vi "SMU Switch Handshaking - Advanced - DMM- RT.vi"(8 "error in":errorcluster, 11 "file path (use dialog)":path=path "C:/jsontestfile.json") -> (0 "error out":errorcluster, 2 "Results":T1)   [LabVIEW 2019]
uses:
  <instrlib>/niSwitch/niSwitch.llb/niSwitch Topologies.ctl
  <instrlib>/niSwitch/niSwitch.llb/niSwitch Trigger Input.ctl
  <instrlib>/niSwitch/niSwitch.llb/niSwitch Scan Advanced Output.ctl
  <instrlib>/niDMM/nidmm.llb/niDMM Function.ctl
  <instrlib>/niDMM/nidmm.llb/niDMM Trigger.ctl
  <instrlib>/niDMM/nidmm.llb/niDMM Slope.ctl
  Results.ctl
  <instrlib>/niDCPower/nidcpower.llb/niDCPower Export Signal - Signal.ctl
  <instrlib>/niDMM/nidmm.llb/niDMM Sample Trigger.ctl
  <instrlib>/niDMM/nidmm.llb/niDMM Control Actions.ctl
  <instrlib>/niDCPower/nidcpower.llb/niDCPower Wait For Event - Event.ctl
  <instrlib>/niDMM/nidmm.llb/niDMM Configure Measurement Absolute.vi
  <instrlib>/niDCPower/nidcpower.llb/niDCPower Configure Digital Edge Start Trigger.vi
  <instrlib>/niDCPower/nidcpower.llb/niDCPower Configure Digital Edge Sequence Advance Trigger.vi
  <vilib>/ptbypt/NI_PtbyPt.lvlib
panel:
  out "Results":dbl[][](array[numeric])
  out "R ch5 Array":dbl[](array[numeric])
  out "R ch4 Array":dbl[](array[numeric])
  out "R ch3 Array":dbl[](array[numeric])
  out "R ch2 Array":dbl[](array[numeric])
  out "R ch1 Array":dbl[](array[numeric])
  out "R ch0 Array":dbl[](array[numeric])
  out "JSON String":string="{\n    \"resourceName\": \"SMU\",\n    \"channels\": \"0\",\n    \"sourceTransientResponse\": 1039,\n    \"current\": 0.1,\n    \"currentLevelRange\": 0.1,\n    \"measurementSense\": 1008,\n    \"measurementApertureTime\": 0.0833333,\n    \"sourceAdvancedSourceDelay\": 0.000040,\n    \"voltage\": 0.6,\n    \"sourceAdvancedSequenceLoopCount\": 39,\n    \"measurementAdvancedDCNoiseRejection\": 1044    \n}"
  in  "JSON String":string="{\n    \"resourceName\": \"SMU\",\n    \"channels\": \"0\",\n    \"sourceTransientResponse\": 1039,\n    \"current\": 0.1,\n    \"currentLevelRange\": 0.1,\n    \"measurementSense\": 1008,\n    \"measurementApertureTime\": 0.0833333,\n    \"sourceAdvancedSourceDelay\": 0.000040,\n    \"voltage\": 0.6,\n    \"sourceAdvancedSequenceLoopCount\": 39,\n    \"measurementAdvancedDCNoiseRejection\": 1044    \n}"
  in  "Cluster":T2
  out "R ch5":dbl=-61.88328365962959 format="%#_8p"
  out "Waveform Chart ch5":dbl(graph)=-61.88328365962959
  out "standard deviation ch5":dbl=51.51492223632956 format="%.6p"
  out "R ch2":dbl=68.72185379555 format="%#_8p"
  out "Waveform Chart ch2":dbl(graph)=68.72185379555
  out "standard deviation ch2":dbl=53.289896328860735 format="%.6p"
  out "R ch4":dbl=32.16858920728009 format="%#_8p"
  out "Waveform Chart ch4":dbl(graph)=32.16858920728009
  out "standard deviation ch4":dbl=125.6401985791479 format="%.6p"
  out "R ch1":dbl=60.088322199824006 format="%#_8p"
  out "Waveform Chart ch1":dbl(graph)=60.088322199824006
  out "standard deviation ch1":dbl=77.80595142647893 format="%.6p"
  out "R ch3":dbl=-18.415997181850322 format="%#_8p"
  out "Waveform Chart ch3":dbl(graph)=-18.415997181850322
  out "standard deviation ch3":dbl=58.115118389377486 format="%.6p"
  out "standard deviation ch0":dbl=nan format="%.6p"
  out "Waveform Chart ch0":dbl(graph)=-33.87929256021835
  out "R ch0":dbl=-33.87929256021835 format="%#_8p"
  out "voltage measurements":dbl[](array[numeric])=[8.973959484137595e-05, 8.72183300089091e-05, 8.719984907656908e-05]
  in  "Configuration:Advanced:Number Of Averages":i32=1
  in  "Configuration:Advanced:Aperture Time":dbl=0.05
  in  "Configuration:Advanced:Aperture Time Units":i32(ring) items=["Seconds", "Power Line Cycles"]
  in  "Device Name":refnum<k15>="DMM"
  in  "Slope":T3
  in  "DMM Trigger Source":T4=enum."TTL 2"
  in  "Range":dbl=0.1 format="%.2p"
  in  "Function":T5
  out "Elapsed Time (ms)":u32=11998
  in  "scan advanced output (External)":T6=enum."TTL1" caption="Scan Advanced Destination"
  in  "Trigger Source":T7=enum."TTL0"
  in  "topology name":T8="2527/4-Wire 16x1 Mux" caption="Topology Name"
  in  "scan list":string="ch0:5->com0;\n" caption="Scan List"
  in  "resource name 2":refnum<k15>="2527" caption="Switch Resource Name"
  out "current measurements":dbl[](array[numeric])=[-3.1718829630035887e-06, -3.2085709260490515e-06, -3.2269149075717425e-06]
  in  "resource name":refnum<k15>="SMU" caption="SMU resource name"
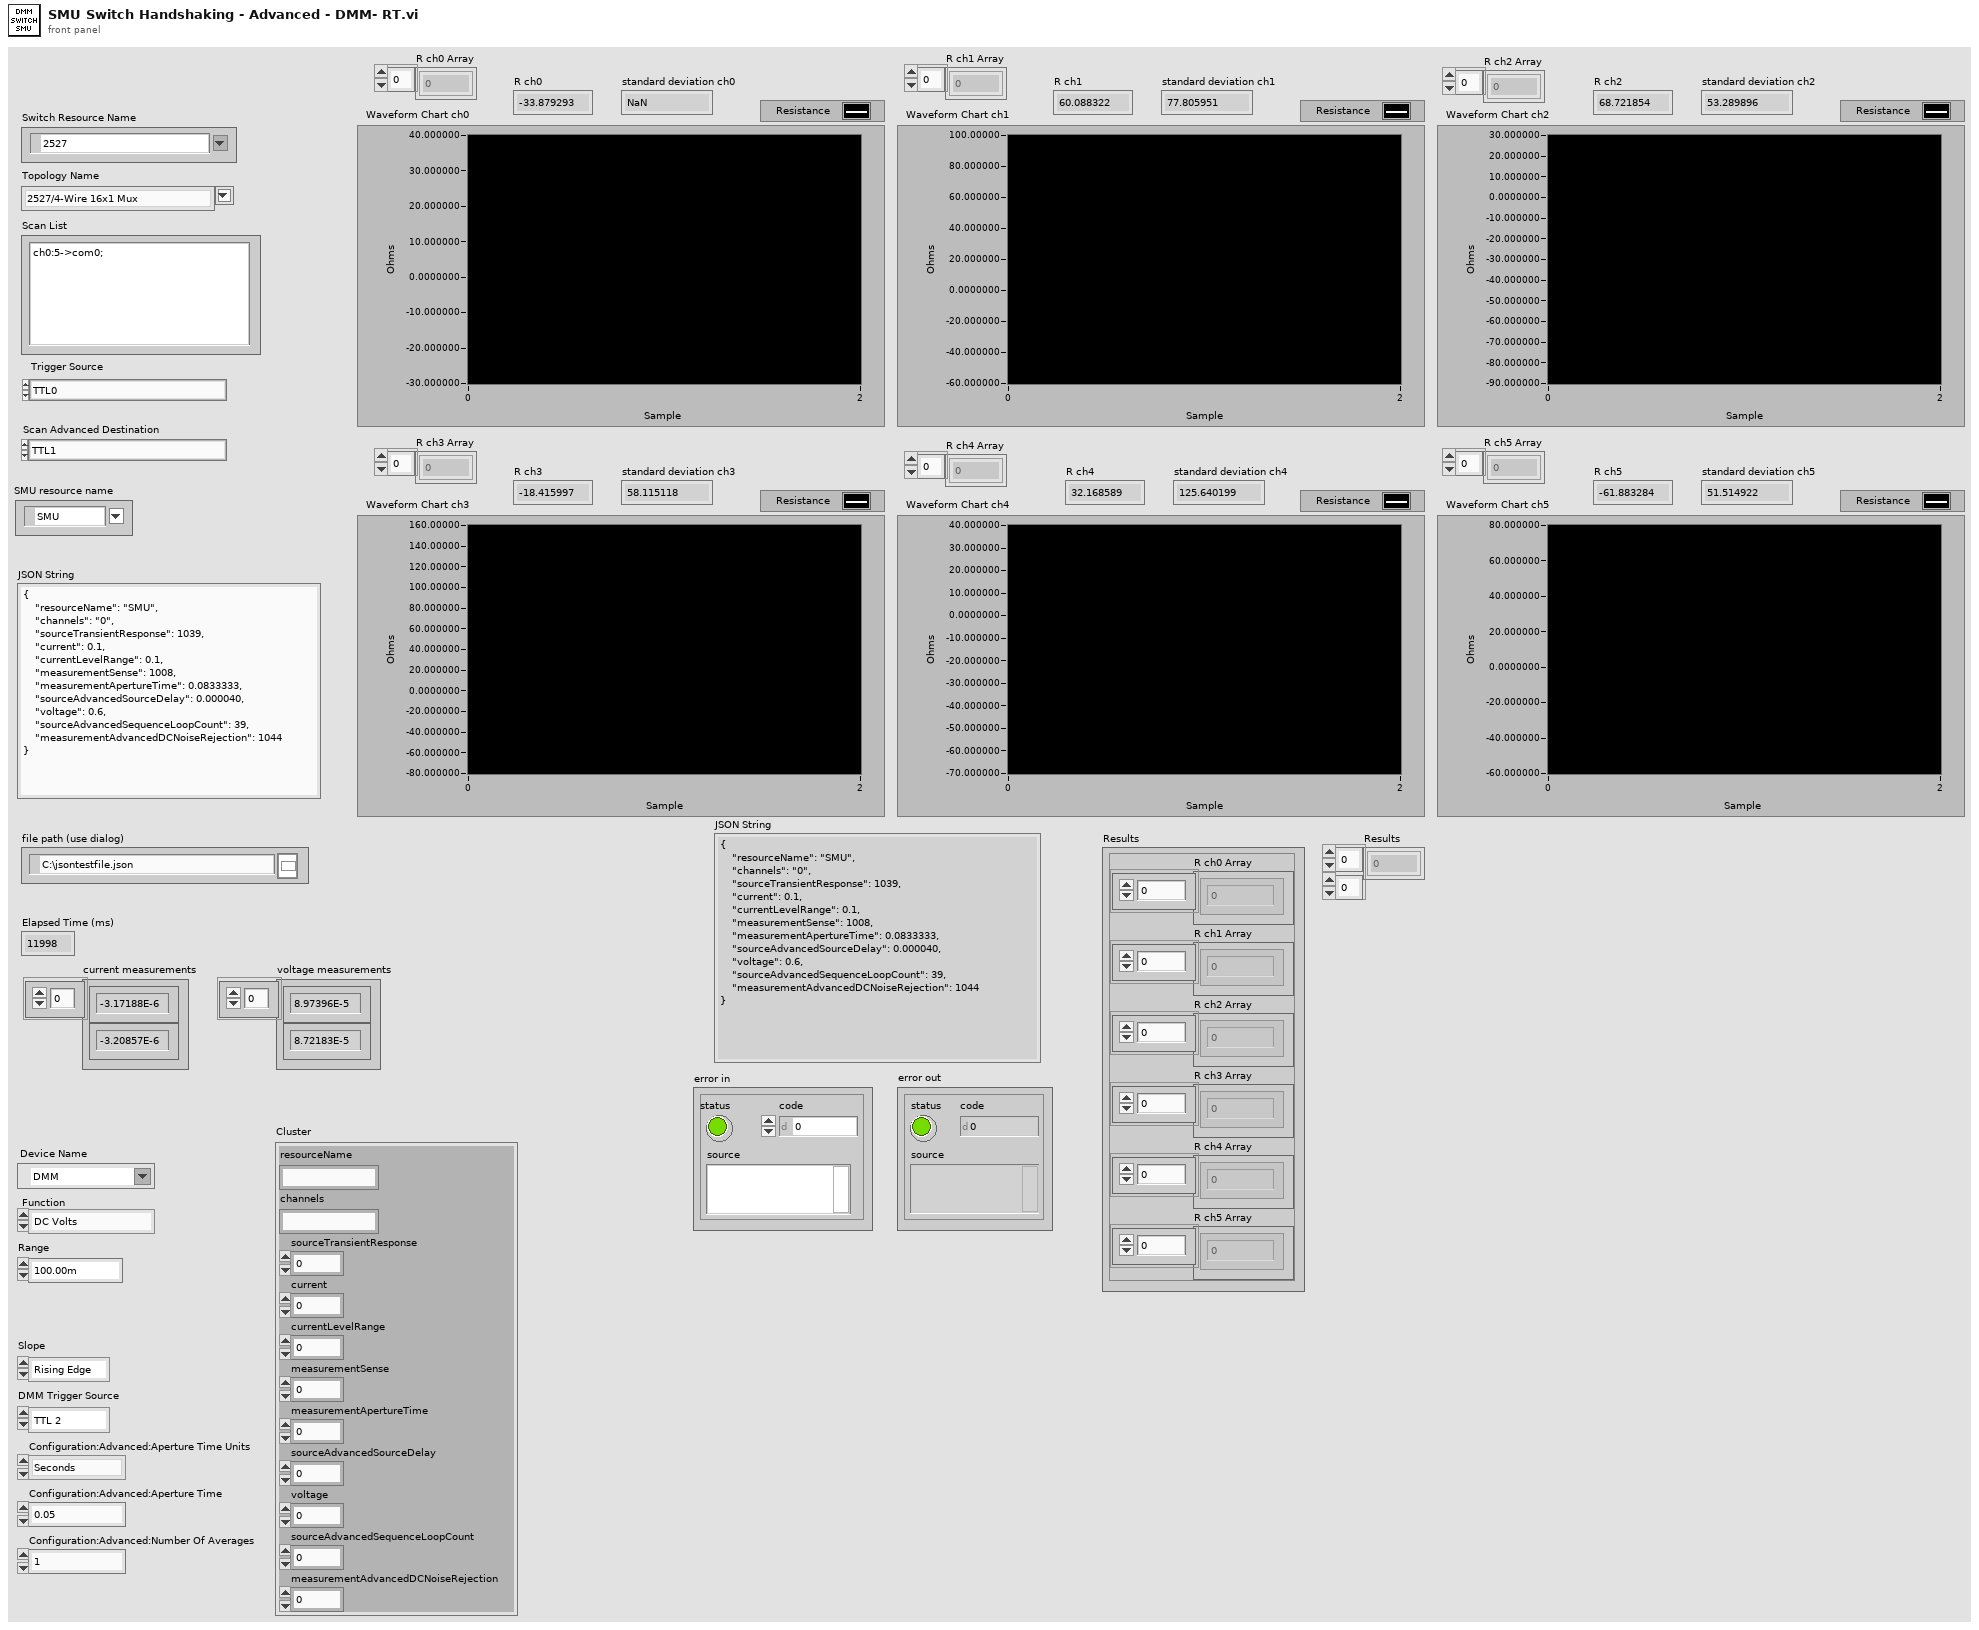
[diagram p1: front panel]
types:
  T1 = typedef "Results.ctl" = cluster{"R ch0 Array":dbl[], "R ch1 Array":dbl[], "R ch2 Array":dbl[], "R ch3 Array":dbl[], "R ch4 Array":dbl[], "R ch5 Array":dbl[]}
  T2 = cluster{"resourceName":string, "channels":string, "sourceTransientResponse":i32, "current":dbl, "currentLevelRange":dbl, "measurementSense":i32, "measurementApertureTime":dbl, "sourceAdvancedSourceDelay":dbl, "voltage":dbl, "sourceAdvancedSequenceLoopCount":i32, "measurementAdvancedDCNoiseRejection":i32}
  T3 = typedef "niDMM Slope.ctl" = enum16{"Rising Edge", "Falling Edge"}
  T4 = typedef "niDMM Trigger.ctl" = enum16{"Immediate", "External", "TTL 0", "TTL 1", "TTL 2", "TTL 3", "TTL 4", "TTL 5", "TTL 6", "Software", "TTL 7", "PXI Star", "LBR Trig 1", "Aux Trig 1"}
  T5 = typedef "niDMM Function.ctl" = enum16{"DC Volts", "AC Volts", "DC Current", "AC Current", "2-wire Resistance", "4-wire Resistance", "Diode", "Frequency", "Period", "AC Volts DC Coupled", "Capacitance", "Inductance", "Temperature"}
  T6 = typedef "niSwitch Scan Advanced Output.ctl" = enum16{"None", "External", "TTL0", "TTL1", "TTL2", "TTL3", "TTL4", "TTL5", "TTL6", "TTL7", "ECL0", "ECL1", "PXI Star", "Rear Connector", "Front Connector", "Rear Connector Module 1", "Rear Connector Module 2", "Rear Connector Module 3", "Rear Connector Module 4", "Rear Connector Module 5", "Rear Connector Module 6", "Rear Connector Module 7", "Rear Connector Module 8", "Rear Connector Module 9", "Rear Connector Module 10", "Rear Connector Module 11", "Rear Connector Module 12", "Front Connector Module 1", "Front Connector Module 2", "Front Connector Module 3", "Front Connector Module 4", "Front Connector Module 5", "Front Connector Module 6", "Front Connector Module 7", "Front Connector Module 8", "Front Connector Module 9", "Front Connector Module 10", "Front Connector Module 11", "Front Connector Module 12"}
  T7 = typedef "niSwitch Trigger Input.ctl" = enum16{"Immediate", "External", "TTL0", "TTL1", "TTL2", "TTL3", "TTL4", "TTL5", "TTL6", "TTL7", "ECL0", "ECL1", "PXI Star", "Software Trigger Function", "Rear Connector", "Front Connector", "Rear Connector of Module 1", "Rear Connector of Module 2", "Rear Connector of Module 3", "Rear Connector of Module 4", "Rear Connector of Module 5", "Rear Connector of Module 6", "Rear Connector of Module 7", "Rear Connector of Module 8", "Rear Connector of Module 9", "Rear Connector of Module 10", "Rear Connector of Module 11", "Rear Connector of Module 12", "Front Connector of Module 1", "Front Connector of Module 2", "Front Connector of Module 3", "Front Connector of Module 4", "Front Connector of Module 5", "Front Connector of Module 6", "Front Connector of Module 7", "Front Connector of Module 8", "Front Connector of Module 9", "Front Connector of Module 10", "Front Connector of Module 11", "Front Connector of Module 12"}
  T8 = typedef "niSwitch Topologies.ctl" = string
  T9 = enum16{"open", "replace", "create", "open or create", "replace or create", "replace or create with confirmation"}
  T10 = typedef "niDCPower Export Signal - Signal.ctl" = i32
  T11 = typedef "niDMM Control Actions.ctl" = i32
  T12 = typedef "niDMM Sample Trigger.ctl" = enum16{"Immediate", "External", "TTL 0", "TTL 1", "TTL 2", "TTL 3", "TTL 4", "TTL 5", "TTL 6", "Interval", "Software", "TTL 7", "PXI Star", "LBR Trig 1", "Aux Trig 1"}
  T13 = typedef "niDCPower Wait For Event - Event.ctl" = i32
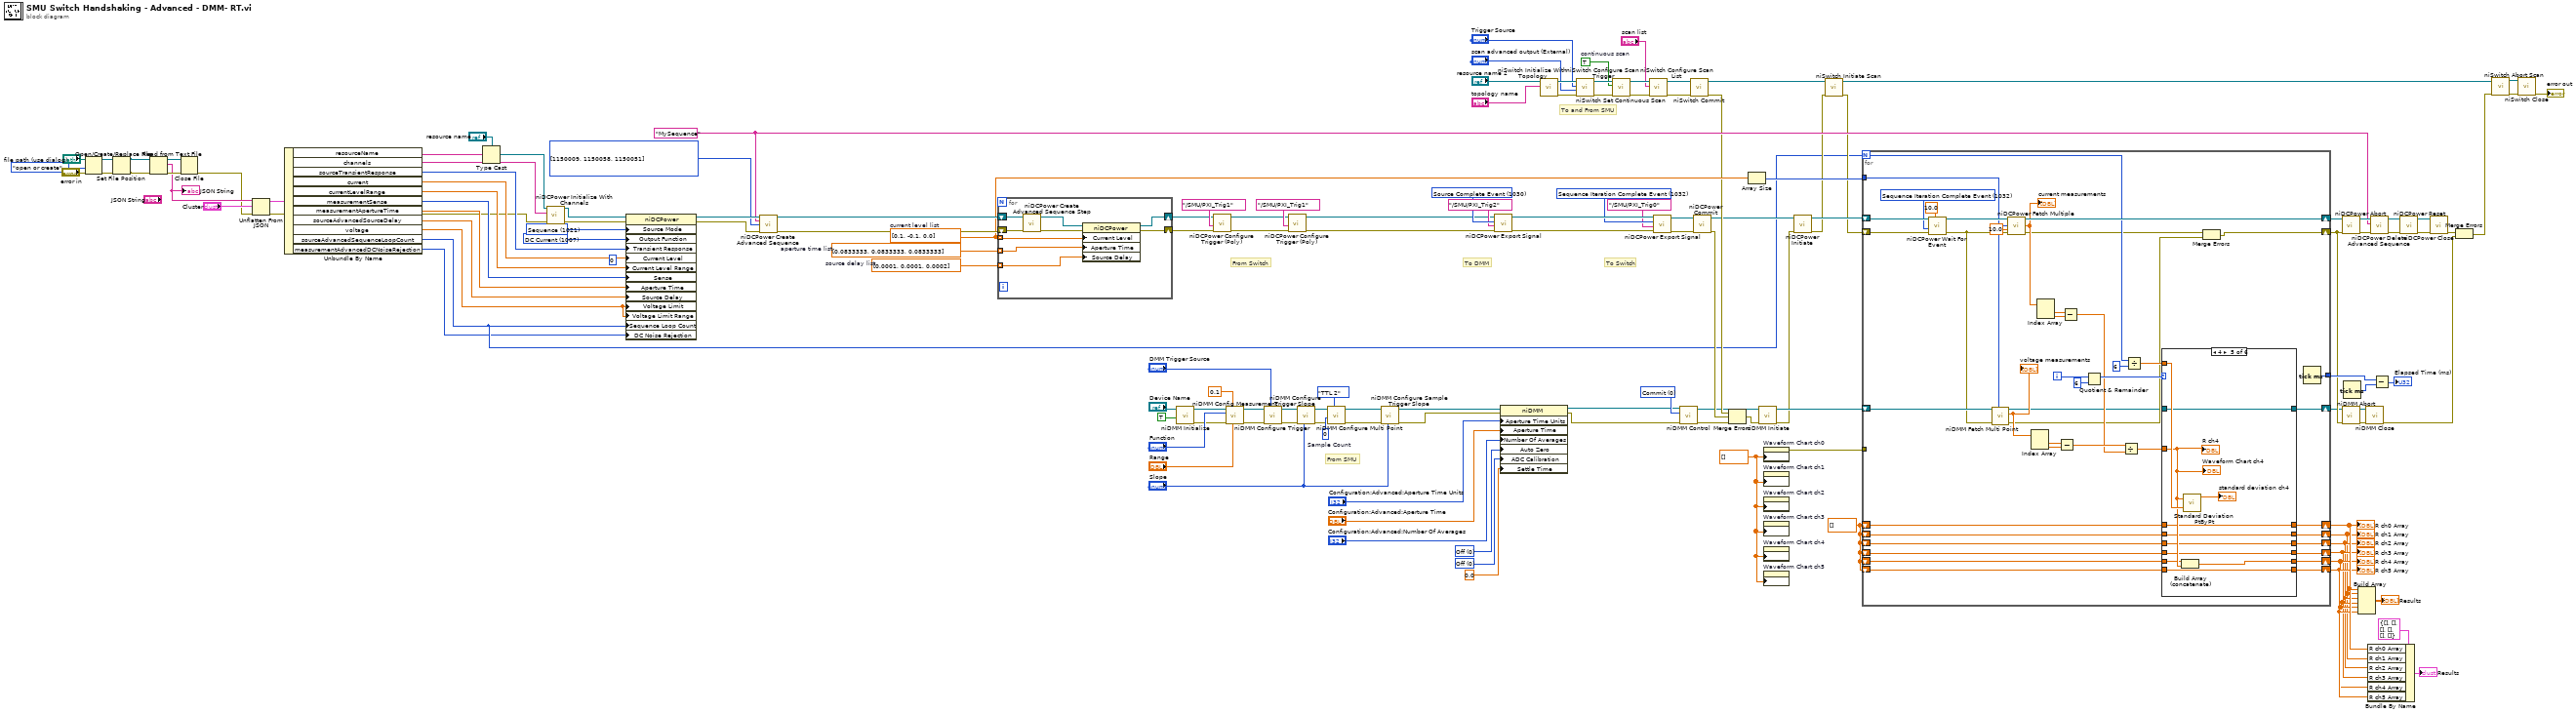
[diagram p0: block diagram]
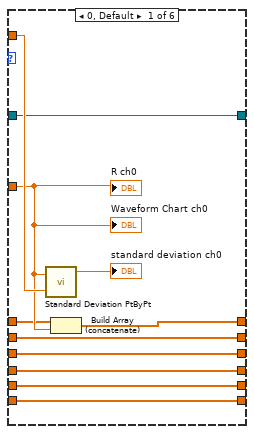
[diagram p2: hidden frame]
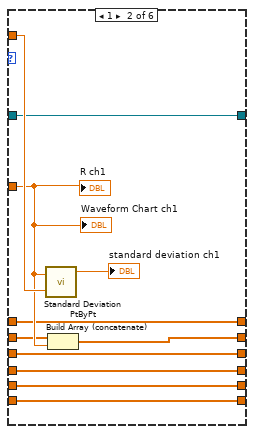
[diagram p3: hidden frame]
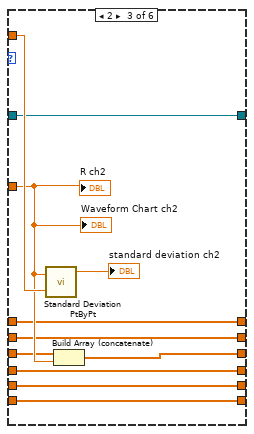
[diagram p4: hidden frame]
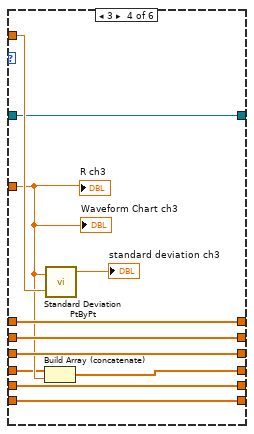
[diagram p5: hidden frame]
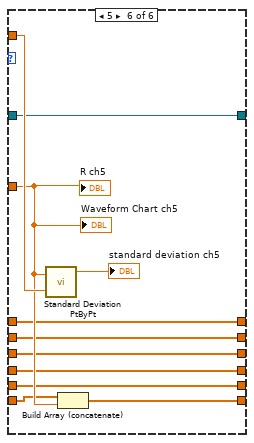
[diagram p6: hidden frame]
diagram:
  w10 = dbl[] []
  (unwired) 0 ("sourceTransientResponse")
  w39 = 0 items=["Auto"=-1, "Off"=0, "On"=1] ("Configuration:Measurement Options:ADC Calibration")
  w40 = 0 items=["Auto"=-1, "Off"=0, "On"=1, "Once"=2] ("Configuration:Measurement Options:Auto Zero")
  w44 = T10 1032 items=["Source Complete Event"=1030, "Measure Complete Event"=1031, "Sequence Iteration Complete Event"=1032, "Sequence Engine Done Event"=1033, "Pulse Complete Event"=1051, "Ready For Pulse Trigger Event"=1052, "Start Trigger"=1034, "Source Trigger"=1035, "Measure Trigger"=1036, "Sequence Advance Trigger"=1037, "Pulse Trigger"=1053] ("signal")
  w68 = T11 0 items=["Commit"] ("Control Action")
  w90 = 0  # Sample Count
  w95 = T10 1030 items=["Source Complete Event"=1030, "Measure Complete Event"=1031, "Sequence Iteration Complete Event"=1032, "Sequence Engine Done Event"=1033, "Pulse Complete Event"=1051, "Ready For Pulse Trigger Event"=1052, "Start Trigger"=1034, "Source Trigger"=1035, "Measure Trigger"=1036, "Sequence Advance Trigger"=1037, "Pulse Trigger"=1053] ("signal")
  w98 = dbl[] [0.1, -0.1, 0.0]  # current level list
  w45 = dbl[] [0.0833333, 0.0833333, 0.0833333]  # aperture time list
  w104 = i32[] [1150009, 1150058, 1150051] items=["Source -> Output Function"=1150008, "Source -> Output Enabled"=1250006, "Source -> Output Resistance"=1150061, "Source -> Transient Response"=1150062, "Source -> Custom Transient Response -> Voltage Gain Bandwidth"=1150067, "Source -> Custom Transient Response -> Voltage Compensation Frequency"=1150068, "Source -> Custom Transient Response -> Voltage Pole-Zero Ratio"=1150069, "Source -> Custom Transient Response -> Current Gain Bandwidth"=1150070, "Source -> Custom Transient Response -> Current Compensation Frequency"=1150071, "Source -> Custom Transient Response -> Current Pole-Zero Ratio"=1150072, "Source -> DC Voltage -> Voltage Level"=1250001, "Source -> DC Voltage -> Voltage Level Range"=1150005, "Source -> DC Voltage -> Current Limit"=1250005, "Source -> DC Voltage -> Current Limit High"=1150187, "Source -> DC Voltage -> Current Limit Low"=1150188, "Source -> DC Voltage -> Current Limit Range"=1150004, "Source -> DC Current -> Current Level"=1150009, "Source -> DC Current -> Current Level Range"=1150011, "Source -> DC Current -> Voltage Limit"=1150010, "Source -> DC Current -> Voltage Limit High"=1150185, "Source -> DC Current -> Voltage Limit Low"=1150186, "Source -> DC Current -> Voltage Limit Range"=1150012, "Source -> Pulse Voltage -> Pulse Voltage Level"=1150080, "Source -> Pulse Voltage -> Pulse Bias Voltage Level"=1150082, "Source -> Pulse Voltage -> Pulse Voltage Level Range"=1150084, "Source -> Pulse Voltage -> Pulse Current Limit"=1150081, "Source -> Pulse Voltage -> Pulse Current Limit High"=1150193, "Source -> Pulse Voltage -> Pulse Current Limit Low"=1150194, "Source -> Pulse Voltage -> Pulse Bias Current Limit"=1150083, "Source -> Pulse Voltage -> Pulse Bias Current Limit High"=1150195, "Source -> Pulse Voltage -> Pulse Bias Current Limit Low"=1150196, "Source -> Pulse Voltage -> Pulse Current Limit Range"=1150085, "Source -> Pulse Current -> Pulse Current Level"=1150086, "Source -> Pulse Current -> Pulse Bias Current Level"=1150088, "Source -> Pulse Current -> Pulse Current Level Range"=1150090, "Source -> Pulse Current -> Pulse Voltage Limit"=1150087, "Source -> Pulse Current -> Pulse Voltage Limit High"=1150189, "Source -> Pulse Current -> Pulse Voltage Limit Low"=1150190, "Source -> Pulse Current -> Pulse Bias Voltage Limit"=1150089, "Source -> Pulse Current -> Pulse Bias Voltage Limit High"=1150191, "Source -> Pulse Current -> Pulse Bias Voltage Limit Low"=1150192, "Source -> Pulse Current -> Pulse Voltage Limit Range"=1150091, "Source -> Advanced -> Source Delay"=1150051, "Source -> Advanced -> Pulse Bias Delay"=1150092, "Source -> Advanced -> Pulse On Time"=1150093, "Source -> Advanced -> Pulse Off Time"=1150094, "Source -> Advanced -> OVP Enabled"=1250002, "Source -> Advanced -> OVP Limit"=1250003, "Source -> Advanced -> Compliance Limit Symmetry"=1150184, "Source -> Advanced -> Sequence Step Delta Time"=1150198, "Measurement -> Sense"=1150013, "Measurement -> Aperture Time"=1150058, "Measurement -> Measure Record Length"=1150063, "Measurement -> Advanced -> DC Noise Rejection"=1150066] ("advanced sequence properties")
  w105 = "MySequence" ("sequence name")
  w136 = TRUE  # continuous scan
  w101 = dbl[] [0.0001, 0.0001, 0.0002]  # source delay list
  w48 = dbl[] [] ("History Data")
  w145 = 1007 items=["DC Voltage"=1006, "DC Current"=1007, "Pulse Voltage"=1049, "Pulse Current"=1050] ("Source:Output Function")
  w146 = 1021 items=["Single Point"=1020, "Sequence"=1021] ("Source:Source Mode")
  # "To and From SMU"
  # "From SMU"
  # "To Switch"
  # "To DMM"
  # "From Switch"
  n1 = Open/Create/Replace File(file path (use dialog)="file path (use dialog)", error in="error in", operation (0:open)=T9."open or create") -> (refnum out=w16:refnum<file>, error out=w15:errorcluster)  [unwired: 3 in, 1 out]
  n2 = Set File Position(refnum=w16, error in=w15) -> (refnum out=w18:refnum<file>, error out=w17:errorcluster)  [unwired: 2 in]
  n3 = Read from Text File(file (use dialog)=w18, error in=w17) -> (refnum out=w20:refnum<file>, text=w14:string, error out=w19:errorcluster)  [unwired: 2 in, 1 out]
  "JSON String" <- w14
  n4 = Close File(refnum=w20, error in=w19) -> (error out=w13:errorcluster)  [unwired: 1 out]
  n5 = Unflatten From JSON(JSON string=w14, type and defaults="Cluster", error in (no error)=w13) -> (value=w37:T2, error out=w12:errorcluster)  [unwired: 4 in]
  n6 = Unbundle By Name(w37) -> ("resourceName"=w33:string, "channels"=w32:string, "sourceTransientResponse"=w31:i32, "current"=w34:dbl, "currentLevelRange"=w29:dbl, "measurementSense"=w28:i32, "measurementApertureTime"=w27:dbl, "sourceAdvancedSourceDelay"=w26:dbl, "voltage"=w25:dbl, "sourceAdvancedSequenceLoopCount"=w24:i32, "measurementAdvancedDCNoiseRejection"=w23:i32)
  n7 = Type Cast(type="resource name", x=w33) -> (*(type *) &x=w35:refnum<k15>)
  n8 = call <instrlib>:"niDCPower Initialize With Channels.vi"("error in (no error)"=w12, "channels"=w32, "resource name"=w35) -> ("error out"=w142:errorcluster, "instrument handle out"=w143:refnum<k15>)  [unwired: 7 in]
  n9 = property class="niDCPower"(reference=w143, error in=w142, "Source Mode"=w146, "Output Function"=w145, "Transient Response"=w31, "Current Level"=w34, "Current Level Range"=w29, "Sense"=w28, "Aperture Time"=w27, "Source Delay"=w26, "Voltage Limit"=w25, "Voltage Limit Range"=w25, "Sequence Loop Count"=w24, "DC Noise Rejection"=w23) -> (reference out=w113:refnum<k15>, error out=w112:errorcluster)
  n10 = call <instrlib>:"niDCPower Create Advanced Sequence.vi"("instrument handle"=w113, "sequence name"=w105, "advanced sequence properties"=w104, "error in (no error)"=w112) -> ("instrument handle out"=w103:refnum<k15>, "error out"=w102:errorcluster)  [unwired: 10 in]
  n11 = for {
    shift-right: [w152] -> w99
    shift-left: w102 -> [w155]
    shift-right: [w151] -> w100
    shift-left: w103 -> [w150]
    tunnel: w101 -> [w149] mode=indexing
    tunnel: w98 -> [w147] mode=indexing
    tunnel: w45 -> [w148] mode=indexing
    n12 = call <instrlib>:"niDCPower Create Advanced Sequence Step.vi"("error in (no error)"=w155, "instrument handle"=w150) -> ("error out"=w153:errorcluster, "instrument handle out"=w154:refnum<k15>)  [unwired: 8 in]
    n13 = property class="niDCPower"(reference=w154, error in=w153, "Current Level"=w147, "Aperture Time"=w148, "Source Delay"=w149) -> (reference out=w151:refnum<k15>, error out=w152:errorcluster)
  }
  n14 = call <instrlib>:"niDMM Initialize.vi"("Reset"=TRUE, "Instrument Descriptor"="Device Name") -> ("error out"=w76:errorcluster, "instrument handle out"=w75:refnum<k15>)  [unwired: 8 in]
  n15 = call-poly <instrlib>:"niDCPower Configure Trigger (Poly).vi"("error in (no error)"=w99, "input terminal"=tag "/SMU/PXI_Trig1", "instrument handle"=w100) -> ("error out"=w117:errorcluster, "instrument handle out"=w118:refnum<k15>)  [unwired: 7 in]
  n16 = call-poly <instrlib>:"niDMM Config Measurement.vi"("Range"="Range", "Resolution"=0.1, "error in (no error)"=w76, "Function"="Function", "instrument handle"=w75) -> ("error out"=w82:errorcluster, "instrument handle out"=w81:refnum<k15>)  [unwired: 5 in]
  n17 = call <instrlib>:"niDMM Configure Trigger.vi"("Trigger Source"="DMM Trigger Source", "error in (no error)"=w82, "instrument handle"=w81) -> ("error out"=w84:errorcluster, "instrument handle out"=w83:refnum<k15>)  [unwired: 7 in]
  n18 = call-poly <instrlib>:"niDCPower Configure Trigger (Poly).vi"("error in (no error)"=w117, "input terminal"=tag "/SMU/PXI_Trig1", "instrument handle"=w118) -> ("error out"=w46:errorcluster, "instrument handle out"=w47:refnum<k15>)  [unwired: 7 in]
  n19 = call <instrlib>:"niDMM Configure Trigger Slope.vi"("Slope"="Slope", "error in (no error)"=w84, "instrument handle"=w83) -> ("error out"=w86:errorcluster, "instrument handle out"=w85:refnum<k15>)  [unwired: 7 in]
  n20 = call <instrlib>:"niDMM Configure Multi Point.vi"("Sample Trigger"=niDMM_Sample_Trigger."TTL 2", "error in (no error)"=w86, "Sample Count"=w90, "instrument handle"=w85) -> ("error out"=w88:errorcluster, "instrument handle out"=w87:refnum<k15>)  [unwired: 6 in]
  n21 = call <instrlib>:"niDMM Configure Sample Trigger Slope.vi"("Slope"="Slope", "error in (no error)"=w88, "instrument handle"=w87) -> ("error out"=w59:errorcluster, "instrument handle out"=w60:refnum<k15>)  [unwired: 7 in]
  n22 = call <instrlib>:"niDCPower Export Signal.vi"("error in (no error)"=w46, "output terminal"=tag "/SMU/PXI_Trig2", "signal"=w95, "instrument handle"=w47) -> ("error out"=w96:errorcluster, "instrument handle out"=w97:refnum<k15>)  [unwired: 6 in]
  n23 = property class="niDMM"(reference=w60, error in=w59, "Aperture Time Units"="Configuration:Advanced:Aperture Time Units", "Aperture Time"="Configuration:Advanced:Aperture Time", "Number Of Averages"="Configuration:Advanced:Number Of Averages", "Auto Zero"=w40, "ADC Calibration"=w39, "Settle Time"=0.0 ("Configuration:Advanced:Settle Time")) -> (reference out=w50:refnum<k15>, error out=w49:errorcluster)
  n24 = call <instrlib>:"niSwitch Initialize With Topology.vi"("topology name"="topology name", "resource name"="resource name 2") -> ("error out"=w133:errorcluster, "instrument handle out"=w134:refnum<k15>)  [unwired: 3 in, 5 out]
  n25 = call <instrlib>:"niSwitch Configure Scan Trigger.vi"("error in (no error)"=w133, "scan advanced output (External)"="scan advanced output (External)", "trigger input (External)"="Trigger Source", "instrument handle"=w134) -> ("error out"=w137:errorcluster, "instrument handle out"=w139:refnum<k15>)  [unwired: 1 in, 5 out]
  n26 = call <instrlib>:"niSwitch Set Continuous Scan.vi"("error in (no error)"=w137, "continuous scan (False)"=w136, "instrument handle"=w139) -> ("error out"=w131:errorcluster, "instrument handle out"=w132:refnum<k15>)  [unwired: 7 out]
  n27 = call <instrlib>:"niSwitch Configure Scan List.vi"("error in (no error)"=w131, "scan list"="scan list", "instrument handle"=w132) -> ("error out"=w128:errorcluster, "instrument handle out"=w127:refnum<k15>)  [unwired: 1 in, 6 out]
  n28 = call <instrlib>:"niDCPower Export Signal.vi"("error in (no error)"=w96, "output terminal"=tag "/SMU/PXI_Trig0", "signal"=w44, "instrument handle"=w97) -> ("error out"=w71:errorcluster, "instrument handle out"=w72:refnum<k15>)  [unwired: 6 in]
  n29 = call <instrlib>:"niDMM Control.vi"("error in (no error)"=w49, "Control Action"=w68, "instrument handle"=w50) -> ("error out"=w67:errorcluster, "instrument handle out"=w61:refnum<k15>)  [unwired: 7 in]
  n30 = call <instrlib>:"niSwitch Commit.vi"("error in (no error)"=w128, "instrument handle"=w127) -> ("error out"=w70:errorcluster, "instrument handle out"=w126:refnum<k15>)  [unwired: 8 out]
  n31 = call <instrlib>:"niDCPower Commit.vi"("error in (no error)"=w71, "instrument handle"=w72) -> ("error out"=w69:errorcluster, "instrument handle out"=w64:refnum<k15>)  [unwired: 8 in]
  n32 = Merge Errors(w70, w69, w67) -> (w66:errorcluster)
  n33 = Array Size(array=w98) -> (size(s)=w144:i32)
  n34 = call <instrlib>:"niDMM Initiate.vi"("error in (no error)"=w66, "instrument handle"=w61) -> ("error out"=w65:errorcluster, "instrument handle out"=w73:refnum<k15>)  [unwired: 8 in]
  n35 = property on="Waveform Chart ch0" class="WFChart (strict)"("History Data"=w48) -> (error out=w42:errorcluster)  [unwired: 2 in, 1 out]
  n36 = property on="Waveform Chart ch1" class="WFChart (strict)"("History Data"=w48) -> ()  [unwired: 2 in, 2 out]
  n37 = property on="Waveform Chart ch2" class="WFChart (strict)"("History Data"=w48) -> ()  [unwired: 2 in, 2 out]
  n38 = property on="Waveform Chart ch3" class="WFChart (strict)"("History Data"=w48) -> ()  [unwired: 2 in, 2 out]
  n39 = property on="Waveform Chart ch4" class="WFChart (strict)"("History Data"=w48) -> ()  [unwired: 2 in, 2 out]
  n40 = property on="Waveform Chart ch5" class="WFChart (strict)"("History Data"=w48) -> ()  [unwired: 2 in, 2 out]
  n41 = call <instrlib>:"niDCPower Initiate.vi"("error in (no error)"=w65, "instrument handle"=w64) -> ("error out"=w63:errorcluster, "instrument handle out"=w140:refnum<k15>)  [unwired: 8 in]
  n42 = call <instrlib>:"niSwitch Initiate Scan.vi"("error in (no error)"=w63, "instrument handle"=w126) -> ("error out"=w62:errorcluster, "instrument handle out"=w129:refnum<k15>)  [unwired: 8 out]
  n43 = for {
    N: w24 -> [w187]
    tunnel: w144 -> [w181]
    shift-right: [w172] -> w55
    shift-left: w62 -> [w183]
    shift-right: [w194] -> w141
    shift-left: w140 -> [w198]
    tunnel: w42 -> [_]
    tunnel: [w191] -> w116
    shift-right: [w170] -> w51
    shift-left: w73 -> [w182]
    shift-right: [w167] -> w8
    shift-left: w10 -> [w166]
    shift-right: [w165] -> w2
    shift-left: w10 -> [w164]
    shift-right: [w163] -> w3
    shift-left: w10 -> [w162]
    shift-right: [w161] -> w4
    shift-left: w10 -> [w160]
    shift-right: [w159] -> w5
    shift-left: w10 -> [w158]
    shift-right: [w157] -> w6
    shift-left: w10 -> [w156]
    i -> [w190]
    w197 = T13 1032 items=["Source Complete Event"=1030, "Measure Complete Event"=1031, "Sequence Iteration Complete Event"=1032, "Sequence Engine Done Event"=1033, "Pulse Complete Event"=1051, "Ready For Pulse Trigger Event"=1052] ("event")
    n44 = call <instrlib>:"niDCPower Wait For Event.vi"("timeout (sec)"=10.0, "error in (no error)"=w183, "event"=w197, "instrument handle"=w198) -> ("error out"=w169:errorcluster, "instrument handle out"=w195:refnum<k15>)  [unwired: 6 in]
    n45 = call <instrlib>:"niDMM Fetch Multi Point.vi"("Number to Fetch"=w181, "error in (no error)"=w169, "instrument handle"=w182) -> ("error out"=w173:errorcluster, "Measurements"=w175:dbl[], "instrument handle out"=w171:refnum<k15>)  [unwired: 5 in, 1 out]
    "voltage measurements" <- w175
    n46 = call <instrlib>:"niDCPower Fetch Multiple.vi"("instrument handle"=w195, "count (1)"=w181, "timeout (sec)"=10.0, "error in (no error)"=w169) -> ("instrument handle out"=w194:refnum<k15>, "current measurements"=w193:dbl[], "error out"=w174:errorcluster)  [unwired: 6 in, 3 out]
    "current measurements" <- w193
    n47 = Index Array(array=w175) -> (element #1=w180:dbl, element #2=w179:dbl)  [unwired: 2 in]
    n48 = Index Array(array=w193) -> (element #1=w192:dbl, element #2=w184:dbl)  [unwired: 2 in]
    n49 = Subtract(x=w180, y=w179) -> (x-y=w178:dbl)
    n50 = Subtract(x=w192, y=w184) -> (x-y=w177:dbl)
    n51 = Quotient & Remainder(x=w190, y=6) -> (x-y*floor(x/y)=w188:i32)  [unwired: 1 out]
    n52 = Divide(x=w178, y=w177) -> (x/y=w176:dbl)
    n53 = Divide(x=w187, y=6) -> (x/y=w185:dbl)
    n54 = case shown="4" w188 {
      tunnel: w185 -> [w208 w219 w230 w241 w252 w263]
      tunnel: w176 -> [w206 w217 w228 w236 w250 w261]
      tunnel: w171 -> [w207 w218 w229 w240 w251 w262]
      tunnel: [w207 w218 w229 w240 w251 w262] -> w170
      tunnel: [w205 w214 w225 w239 w247 w258] -> w167
      tunnel: w166 -> [w204 w214 w225 w239 w247 w258]
      tunnel: [w203 w216 w224 w238 w246 w257] -> w165
      tunnel: w164 -> [w203 w215 w224 w238 w246 w257]
      tunnel: [w202 w213 w227 w237 w245 w256] -> w163
      tunnel: w162 -> [w202 w213 w226 w237 w245 w256]
      tunnel: [w201 w212 w223 w235 w244 w255] -> w161
      tunnel: w160 -> [w201 w212 w223 w234 w244 w255]
      tunnel: [w200 w211 w222 w233 w249 w254] -> w159
      tunnel: w158 -> [w200 w211 w222 w233 w248 w254]
      tunnel: [w199 w210 w221 w232 w243 w260] -> w157
      tunnel: w156 -> [w199 w210 w221 w232 w243 w259]
      frame 0, Default {
        n55 = call <vilib>:"Standard Deviation PtByPt.vi"("x"=w206, "sample length"=w208) -> ("standard deviation"=→"standard deviation ch0":dbl)  [unwired: 1 in, 2 out]
        n56 = Build Array (concatenate)(w204, w206) -> (w205:dbl[])
        "R ch0" <- w206
        "Waveform Chart ch0" <- w206
      }
      frame 1 {
        n57 = call <vilib>:"Standard Deviation PtByPt.vi"("x"=w217, "sample length"=w219) -> ("standard deviation"=→"standard deviation ch1":dbl)  [unwired: 1 in, 2 out]
        n58 = Build Array (concatenate)(w215, w217) -> (w216:dbl[])
        "R ch1" <- w217
        "Waveform Chart ch1" <- w217
      }
      frame 2 {
        n59 = call <vilib>:"Standard Deviation PtByPt.vi"("x"=w228, "sample length"=w230) -> ("standard deviation"=→"standard deviation ch2":dbl)  [unwired: 1 in, 2 out]
        n60 = Build Array (concatenate)(w226, w228) -> (w227:dbl[])
        "R ch2" <- w228
        "Waveform Chart ch2" <- w228
      }
      frame 3 {
        n61 = Build Array (concatenate)(w234, w236) -> (w235:dbl[])
        n62 = call <vilib>:"Standard Deviation PtByPt.vi"("x"=w236, "sample length"=w241) -> ("standard deviation"=→"standard deviation ch3":dbl)  [unwired: 1 in, 2 out]
        "R ch3" <- w236
        "Waveform Chart ch3" <- w236
      }
      frame 4 {
        n63 = Build Array (concatenate)(w248, w250) -> (w249:dbl[])
        n64 = call <vilib>:"Standard Deviation PtByPt.vi"("x"=w250, "sample length"=w252) -> ("standard deviation"=→"standard deviation ch4":dbl)  [unwired: 1 in, 2 out]
        "R ch4" <- w250
        "Waveform Chart ch4" <- w250
      }
      frame 5 {
        n65 = call <vilib>:"Standard Deviation PtByPt.vi"("x"=w261, "sample length"=w263) -> ("standard deviation"=→"standard deviation ch5":dbl)  [unwired: 1 in, 2 out]
        n66 = Build Array (concatenate)(w259, w261) -> (w260:dbl[])
        "R ch5" <- w261
        "Waveform Chart ch5" <- w261
      }
    }
    n67 = Merge Errors(w174, w173) -> (w172:errorcluster)
    n68 = Tick Count (ms)() -> (millisecond timer value=w191:u32)
  }
  "R ch0 Array" <- w8
  "R ch1 Array" <- w2
  "R ch2 Array" <- w3
  "R ch3 Array" <- w4
  "R ch4 Array" <- w5
  "R ch5 Array" <- w6
  n69 = call <instrlib>:"niDCPower Abort.vi"("error in (no error)"=w55, "instrument handle"=w141) -> ("error out"=w110:errorcluster, "instrument handle out"=w111:refnum<k15>)  [unwired: 8 in]
  n70 = call <instrlib>:"niDMM Abort.vi"("error in (no error)"=w55, "instrument handle"=w51) -> ("error out"=w78:errorcluster, "instrument handle out"=w77:refnum<k15>)  [unwired: 8 in]
  n71 = Tick Count (ms)() -> (millisecond timer value=w115:u32)
  n72 = Build Array(w8, w2, w3, w4, w5, w6) -> (→"Results":dbl[][])
  n73 = call <instrlib>:"niDMM Close.vi"("error in (no error)"=w78, "instrument handle"=w77) -> ("error out"=w54:errorcluster)  [unwired: 9 in]
  n74 = Bundle By Name(cluster=T1 {"R ch0 Array"=[], "R ch1 Array"=[], "R ch2 Array"=[], "R ch3 Array"=[], "R ch4 Array"=[], "R ch5 Array"=[]}, "R ch0 Array"=w8, "R ch1 Array"=w2, "R ch2 Array"=w3, "R ch3 Array"=w4, "R ch4 Array"=w5, "R ch5 Array"=w6) -> (→"Results":T1)
  n75 = call <instrlib>:"niDCPower Delete Advanced Sequence.vi"("error in (no error)"=w110, "sequence name"=w105, "instrument handle"=w111) -> ("error out"=w109:errorcluster, "instrument handle out"=w108:refnum<k15>)  [unwired: 7 in]
  n76 = Subtract(x=w116, y=w115) -> (x-y=→"Elapsed Time (ms)":u32)
  n77 = call <instrlib>:"niDCPower Reset.vi"("error in (no error)"=w109, "instrument handle"=w108) -> ("error out"=w106:errorcluster, "instrument handle out"=w107:refnum<k15>)  [unwired: 2 in, 6 out]
  n78 = call <instrlib>:"niDCPower Close.vi"("error in (no error)"=w106, "instrument handle"=w107) -> ("error out"=w53:errorcluster)  [unwired: 9 in]
  n79 = Merge Errors(w53, w54) -> (w52:errorcluster)
  n80 = call <instrlib>:"niSwitch Abort Scan.vi"("error in (no error)"=w52, "instrument handle"=w129) -> ("error out"=w135:errorcluster, "instrument handle out"=w138:refnum<k15>)  [unwired: 8 out]
  n81 = call <instrlib>:"niSwitch Close.vi"("error in (no error)"=w135, "instrument handle"=w138) -> ("error out"=→"error out":errorcluster)  [unwired: 9 out]
